vi "Get Initialize Edit Sensor.vi"(8 "error in (no error)":errorcluster, 11 "Abstract Initialize Edit Sensor Msg in":refnum<class "Abstract Initialize Edit Sensor Msg.lvclass">) -> (0 "error out":errorcluster, 2 "Initialize Edit Sensor":bool, 3 "Abstract Initialize Edit Sensor Msg out":refnum<class "Abstract Initialize Edit Sensor Msg.lvclass">)   [LabVIEW 2013, in "Edit Sensor Model.lvlib" / "Abstract Initialize Edit Sensor Msg.lvclass"]
uses:
  Abstract Initialize Edit Sensor Msg.lvclass
  Abstract Initialize Edit Sensor Msg.lvclass/Abstract Initialize Edit Sensor Msg.ctl
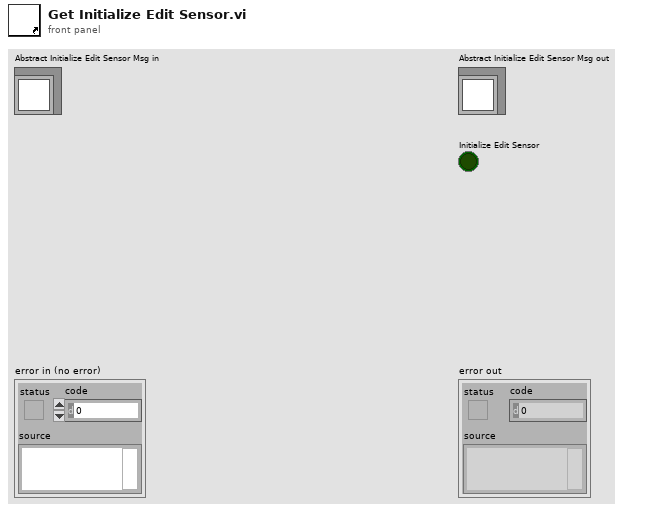
[diagram p1: front panel]
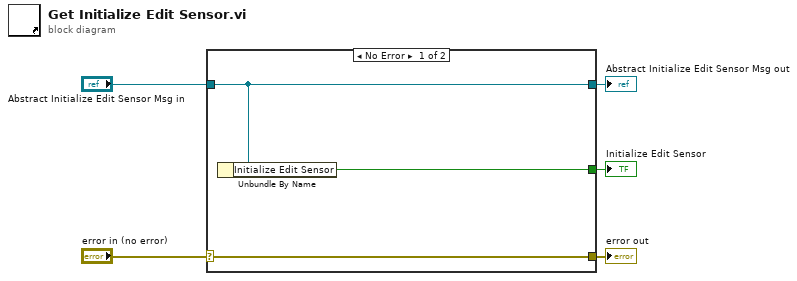
[diagram p0: block diagram]
diagram:
  n1 = case shown="No Error" "error in (no error)" {
    selector: "error in (no error)" -> [w8 w9]
    tunnel: [w8 w9] -> w4
    tunnel: [w7 w10] -> w2
    tunnel: "Abstract Initialize Edit Sensor Msg in" -> [w7 w10]
    tunnel: [w6 _] -> w1
    frame No Error {
      n2 = Unbundle By Name(w7) -> ("Initialize Edit Sensor"=w6:bool)
    }
    frame Error {
    }
  }
  "error out" <- w4
  "Abstract Initialize Edit Sensor Msg out" <- w2
  "Initialize Edit Sensor" <- w1
